vi "getEOTParameters.vi"(8 "error":errorcluster, 10 "axis [0|1|2]":u8, 11 "connection ID":refnum<k5>) -> (0 "error out":errorcluster, 1 "minAvgStepSize_nm":i32, 2 "axis out":u8, 3 "connection ID out":refnum<k5>, 4 "numOfAvgedSteps":i32)   [LabVIEW 2016, in "AMC_VIs.lvlib"]
doc: "This function reads the parameters for the EOT-detection from the device\nInputs:\n -- connection string (from connect_TCP.vi)\n -- axis [0|1|2]\n\nOutputs:\n -- connection ID out\n -- axis out\n -- minAvgStepSize_nm: minimal averaged step-size, that is still not interpreted as eot\n -- numOfAvgedSteps: number of steps, that are averaged to calculate the minAvgStepSize"
uses:
  AMC_VIs.lvlib
panel:
  out "JSON-response":string="{\"jsonrpc\":\"2.0\",\"method\":\"\",\"params\":[5,1.245,true,\"name\"],\"id\":\"1\"}"
  out "JSON request":string
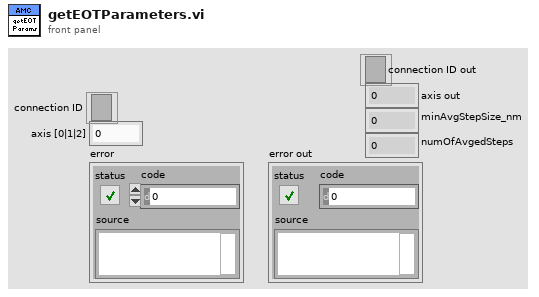
[diagram p1: front panel]
types:
  T1 = cluster{"jsonrpc":string, "method":string, "params":i32[], "id":string, "api":string}
  T2 = cluster{"jsonrpc":string, "result":i32[], "id":string}
  T3 = enum16{"Standard", "Buffered", "CRLF", "Immediate"}
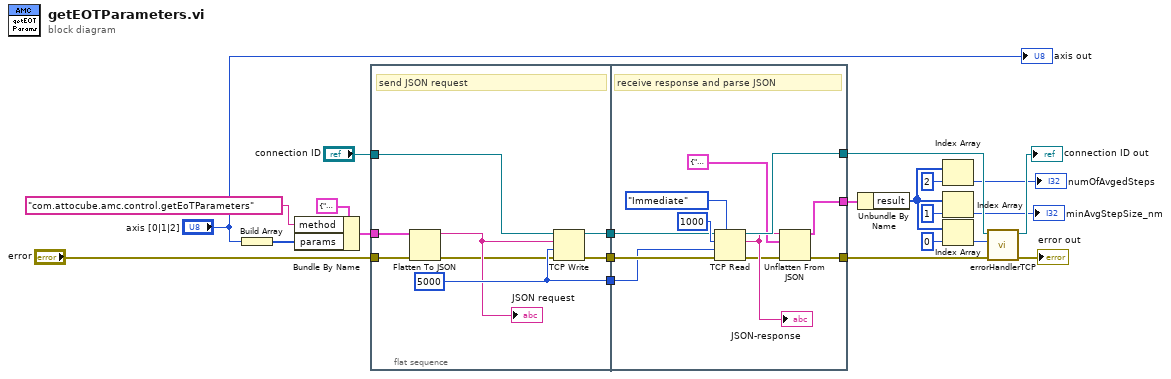
[diagram p0: block diagram]
diagram:
  n1 = Build Array("axis [0|1|2]") -> (w15:u8[])
  n2 = Bundle By Name(cluster=T1 {"jsonrpc"="2.0", "method"="com.attocube.amc.res.setRESReadOutFreq", "params"=[0, 2712], "id"="1", "api"="2"} ("InputParams 2"), "method"="com.attocube.amc.control.getEoTParameters", "params"=w15) -> (w14:T1)
  n3 = flat-sequence {
    tunnel: "connection ID" -> [w30]
    tunnel: [w28] -> w22
    tunnel: [w29] -> w21
    tunnel: "error" -> [w24]
    tunnel: [w27] -> w20
    tunnel: w14 -> [w26]
    tunnel: [w37] -> w7
    tunnel: w22 -> [w39]
    tunnel: w21 -> [w38]
    tunnel: [w33] -> w10
    tunnel: w20 -> [w36]
    tunnel: [w32] -> w13
    frame #0 {
      w27 = 5000 ("timeout ms (25000)")
      # "send JSON request"
      n4 = Flatten To JSON(anything=w26, error in (no error)=w24) -> (JSON string=w25:string, 11:w23:errorcluster)  [unwired: 1 in]
      "JSON request" <- w25
      n5 = TCP Write(connection ID=w30, data in=w25, error in (no error)=w23, 9:w27) -> (connection ID out=w28:refnum<k5>, error out=w29:errorcluster)  [unwired: 1 out]
    }
    frame #1 {
      # "receive response and parse JSON"
      n6 = TCP Read(connection ID=w39, bytes to read=1000, error in (no error)=w38, 7:T3."Immediate" ("mode (standard)"), 9:w36) -> (connection ID out=w37:refnum<k5>, data out=w35:string, error out=w34:errorcluster)
      "JSON-response" <- w35
      n7 = Unflatten From JSON(JSON string=w35, type and defaults=T2 {"jsonrpc"="2.0", "result"=[0, 2712], "id"="1"} ("InputParams 2"), error in (no error)=w34) -> (value=w32:T2, error out=w33:errorcluster)  [unwired: 4 in]
    }
  }
  n8 = Unbundle By Name(w13) -> ("result"=w2:i32[])
  n9 = Index Array(array=w2, index=2) -> (element=→"numOfAvgedSteps":i32)
  n10 = Index Array(array=w2, index=1) -> (element=→"minAvgStepSize_nm":i32)
  n11 = Index Array(array=w2, index=0) -> (element=w9:i32)
  n12 = call "errorHandlerTCP.vi"("error in"=w10, "error number"=w9, "connection ID"=w7) -> ("error out"=→"error out":errorcluster, "connection ID"=→"connection ID out":refnum<k5>)  [unwired: 7 in]
  "axis out" <- "axis [0|1|2]"
